vi "Add Music Element.vi"(8 "error in (no error)":errorcluster, 10 "MusicElement":refnum<class "MusicElement.lvclass">, 11 "MusicElementLibrary in":refnum<class "MusicElementLibrary.lvclass">) -> (0 "error out":errorcluster, 3 "MusicElementLibrary out":refnum<class "MusicElementLibrary.lvclass">)   [LabVIEW 2015, in "MusicElementLibrary.lvclass"]
uses:
  MusicElementLibrary.lvclass
  MusicElement.lvclass
  MusicElementLibrary.lvclass/MusicElementLibrary.ctl
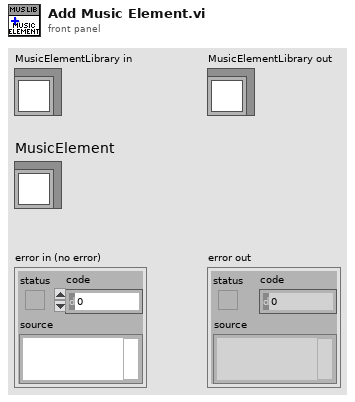
[diagram p1: front panel]
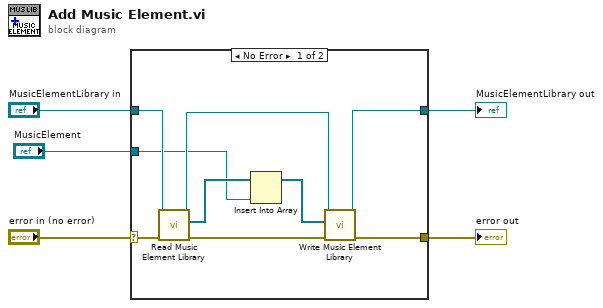
[diagram p0: block diagram]
diagram:
  n1 = case shown="No Error" "error in (no error)" {
    selector: "error in (no error)" -> [w14 w16]
    tunnel: [w8 w16] -> w4
    tunnel: [w9 w15] -> w2
    tunnel: "MusicElementLibrary in" -> [w13 w15]
    tunnel: "MusicElement" -> [w6 _]
    frame No Error {
      n2 = call "Read Music Element Library.vi"("error in (no error)"=w14, "MusicElementLibrary in"=w13) -> ("error out"=w11:errorcluster, "Music Element Library"=w12:refnum<class "MusicElement.lvclass">[], "MusicElementLibrary out"=w10:refnum<class "MusicElementLibrary.lvclass">)  [unwired: 7 in]
      n3 = Insert Into Array(array=w12, new element=w6) -> (w7:refnum<class "MusicElement.lvclass">[])  [unwired: 1 in]
      n4 = call "Write Music Element Library.vi"("error in (no error)"=w11, "Music Element Library"=w7, "MusicElementLibrary in"=w10) -> ("error out"=w8:errorcluster, "MusicElementLibrary out"=w9:refnum<class "MusicElementLibrary.lvclass">)  [unwired: 7 in]
    }
    frame Error {
    }
  }
  "error out" <- w4
  "MusicElementLibrary out" <- w2
